vi "moveTo_abs_XYZ.vi"(7 "blocking?":bool, 8 "error in":errorcluster, 10 "XYZ location (steps)":i32[](array[numeric]), 11 "Actuator cluster in":T1={"Actuator COM"="COM6", "Actuator type"=enum."Scientifica"}) -> (0 "error out":errorcluster, 3 "Actuator cluster out":T1={"Actuator COM"="COM14", "Actuator type"=enum."Scientifica"})   [LabVIEW 2019]
uses:
  controls/actuator_cluster.ctl
  controls/actuator_type.ctl
  controls/scientifica_commands.ctl
panel:
  out "response":string
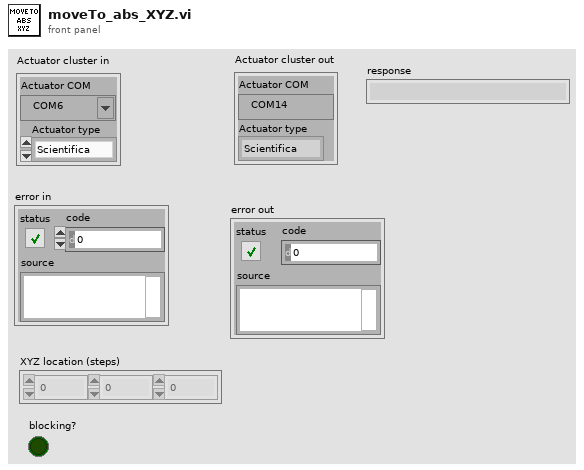
[diagram p1: front panel]
types:
  T1 = typedef "actuator_cluster.ctl" = cluster{"Actuator COM":refnum<visa-resource-name>, "Actuator type":T2}
  T2 = typedef "actuator_type.ctl" = enum16{"Scientifica", "Sutter", "Demo", "Off"}
  T3 = typedef "scientifica_commands.ctl" = enum16{"ANGLE", "INSET", "FIRST", "ZERO", "Pz", "P", "absz", "ACC", "TOP", "STOP", "rel", "relz", "abs", "IN", "vj", "APROACH", "OBJS", "OBJU", "OUT", "OBJ", "OBJL", "SET", "OBJD", "STEP", "SETSTEP", "S", "UUX", "UUY", "UUZ"}
  T4 = enum16{"READY", "ABSOLUTE MOVE", "RELATIVE MOVE", "HOMING", "WAITING", "CANCELING"}
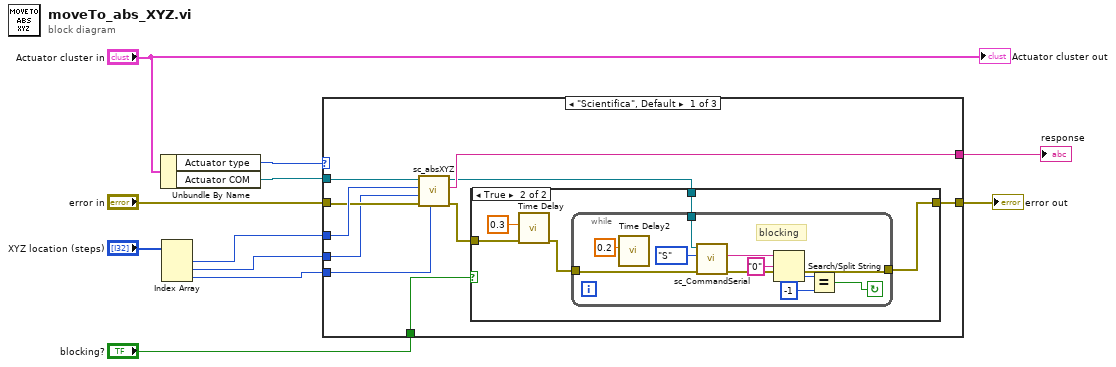
[diagram p0: block diagram]
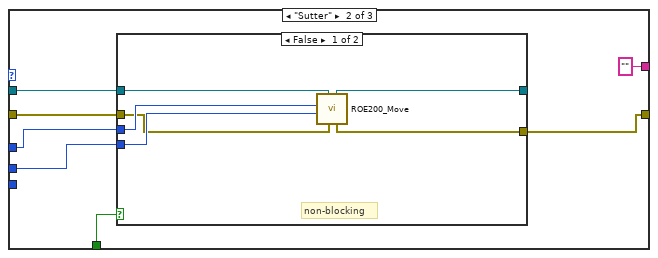
[diagram p3: hidden frame]
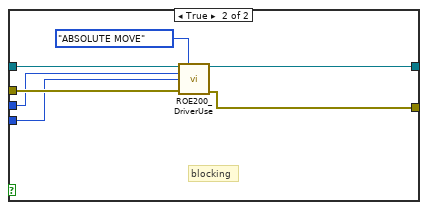
[diagram p4: hidden frame]
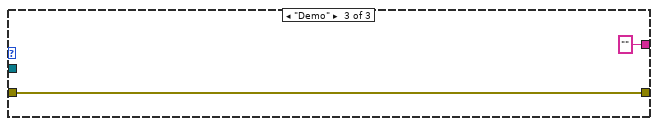
[diagram p5: hidden frame]
diagram:
  n1 = Unbundle By Name("Actuator cluster in") -> ("Actuator type"=w11:T2, "Actuator COM"=w9:refnum<visa-resource-name>)
  n2 = Index Array(array="XYZ location (steps)") -> (element #1=w4:i32, element #2=w3:i32, element #3=w1:i32)  [unwired: 3 in]
  n3 = case shown="\"Scientifica\", Default" w11 {
    tunnel: "error in" -> [w19 w43 w58]
    tunnel: w9 -> [w21 w44 _]
    tunnel: [w14 w39 w58] -> w7
    tunnel: w4 -> [w20 w42 _]
    tunnel: w3 -> [w18 w40 _]
    tunnel: [w17 "" ("argument integer string") "" ("argument integer string")] -> w6
    tunnel: "blocking?" -> [w16 w41 _]
    tunnel: w1 -> [w12 _ _]
    frame "Scientifica", Default {
      n4 = call "sc_absXYZ.vi"("abs Z (steps)"=w12, "error in (no error)"=w19, "abs Y (steps)"=w18, "abs X (steps)"=w20, "VISA handle"=w21) -> ("error out"=w15:errorcluster, "argument integer string"=w17:string, "Dup. VISA handle"=w13:refnum<visa-resource-name>)  [unwired: 4 in]
      n5 = case shown="True" w16 {
        tunnel: w15 -> [w22 w26]
        tunnel: [w22 w24] -> w14
        tunnel: w13 -> [_ w23]
        frame False {
        }
        frame True {
          n6 = call "Time Delay"("error in (no error)"=w26, "Delay Time (s)"=0.3) -> ("error out"=w25:errorcluster)  [unwired: 9 in]
          n7 = while {
            tunnel: w25 -> [w36]
            tunnel: [w30] -> w24
            tunnel: w23 -> [w28]
            stop <- w31 continue-if-true
            # "blocking"
            n8 = call "Time Delay2"("Delay Time (s)"=0.2) -> ()  [unwired: 10 in, 1 out]
            n9 = call "sc_CommandSerial.vi"("error in (no error)"=w36, "Scientifica commands"=scientifica_commands."S", "VISA handle"=w28) -> ("error out"=w30:errorcluster, "Response"=w34:string)  [unwired: 5 in, 2 out]
            n10 = Search/Split String(string=w34, search string/char (-)="0") -> (offset of match=w33:i32)  [unwired: 1 in, 2 out]
            n11 = Equal?(x=w33, y=-1) -> (x = y?=w31:bool)
          }
        }
      }
    }
    frame "Sutter" {
      n12 = case shown="False" w41 {
        tunnel: w44 -> [w50 w57]
        tunnel: w43 -> [w46 w56]
        tunnel: w42 -> [w49 w55]
        tunnel: w40 -> [w48 w54]
        tunnel: [w47 w52] -> _
        tunnel: [w45 w51] -> w39
        frame False {
          # "non-blocking"
          n13 = call "ROE200_Move.vi"("error in (no error)"=w46, "VISA resource name 2"=w50, "Y"=w48, "X"=w49) -> ("error out"=w45:errorcluster, "VISA resource name out"=w47:refnum<visa-resource-name>)  [unwired: 6 in]
        }
        frame True {
          # "blocking"
          n14 = call "ROE200_DriverUse.vi"("VISA resource name In"=w57, "CMD"=T4."ABSOLUTE MOVE", "X"=w55, "Y"=w54, "error in"=w56) -> ("VISA resource name out"=w52:refnum<visa-resource-name>, "error out"=w51:errorcluster)  [unwired: 6 in, 3 out]
        }
      }
    }
    frame "Demo" {
    }
  }
  "error out" <- w7
  "response" <- w6
  "Actuator cluster out" <- "Actuator cluster in"
